vi "offsetZ.vi"(4 "Low Thres":dbl, 6 "Up Thres":dbl, 10 "Current":dbl[][](array[numeric]), 11 "Previous":dbl[][](array[numeric])) -> (2 "OffsetZ":dbl)   [LabVIEW 2011]
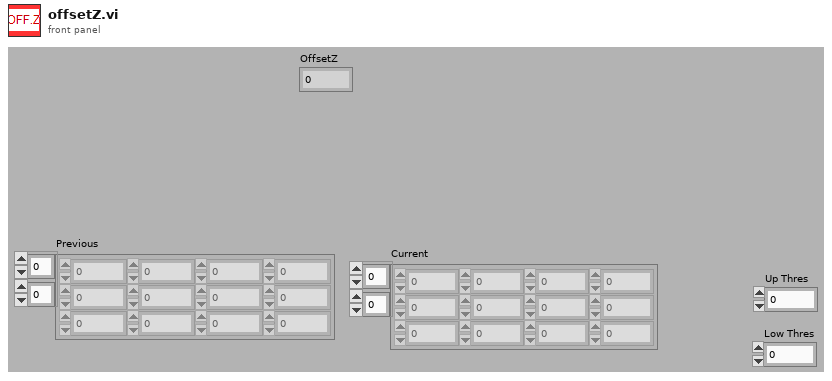
[diagram p1: front panel]
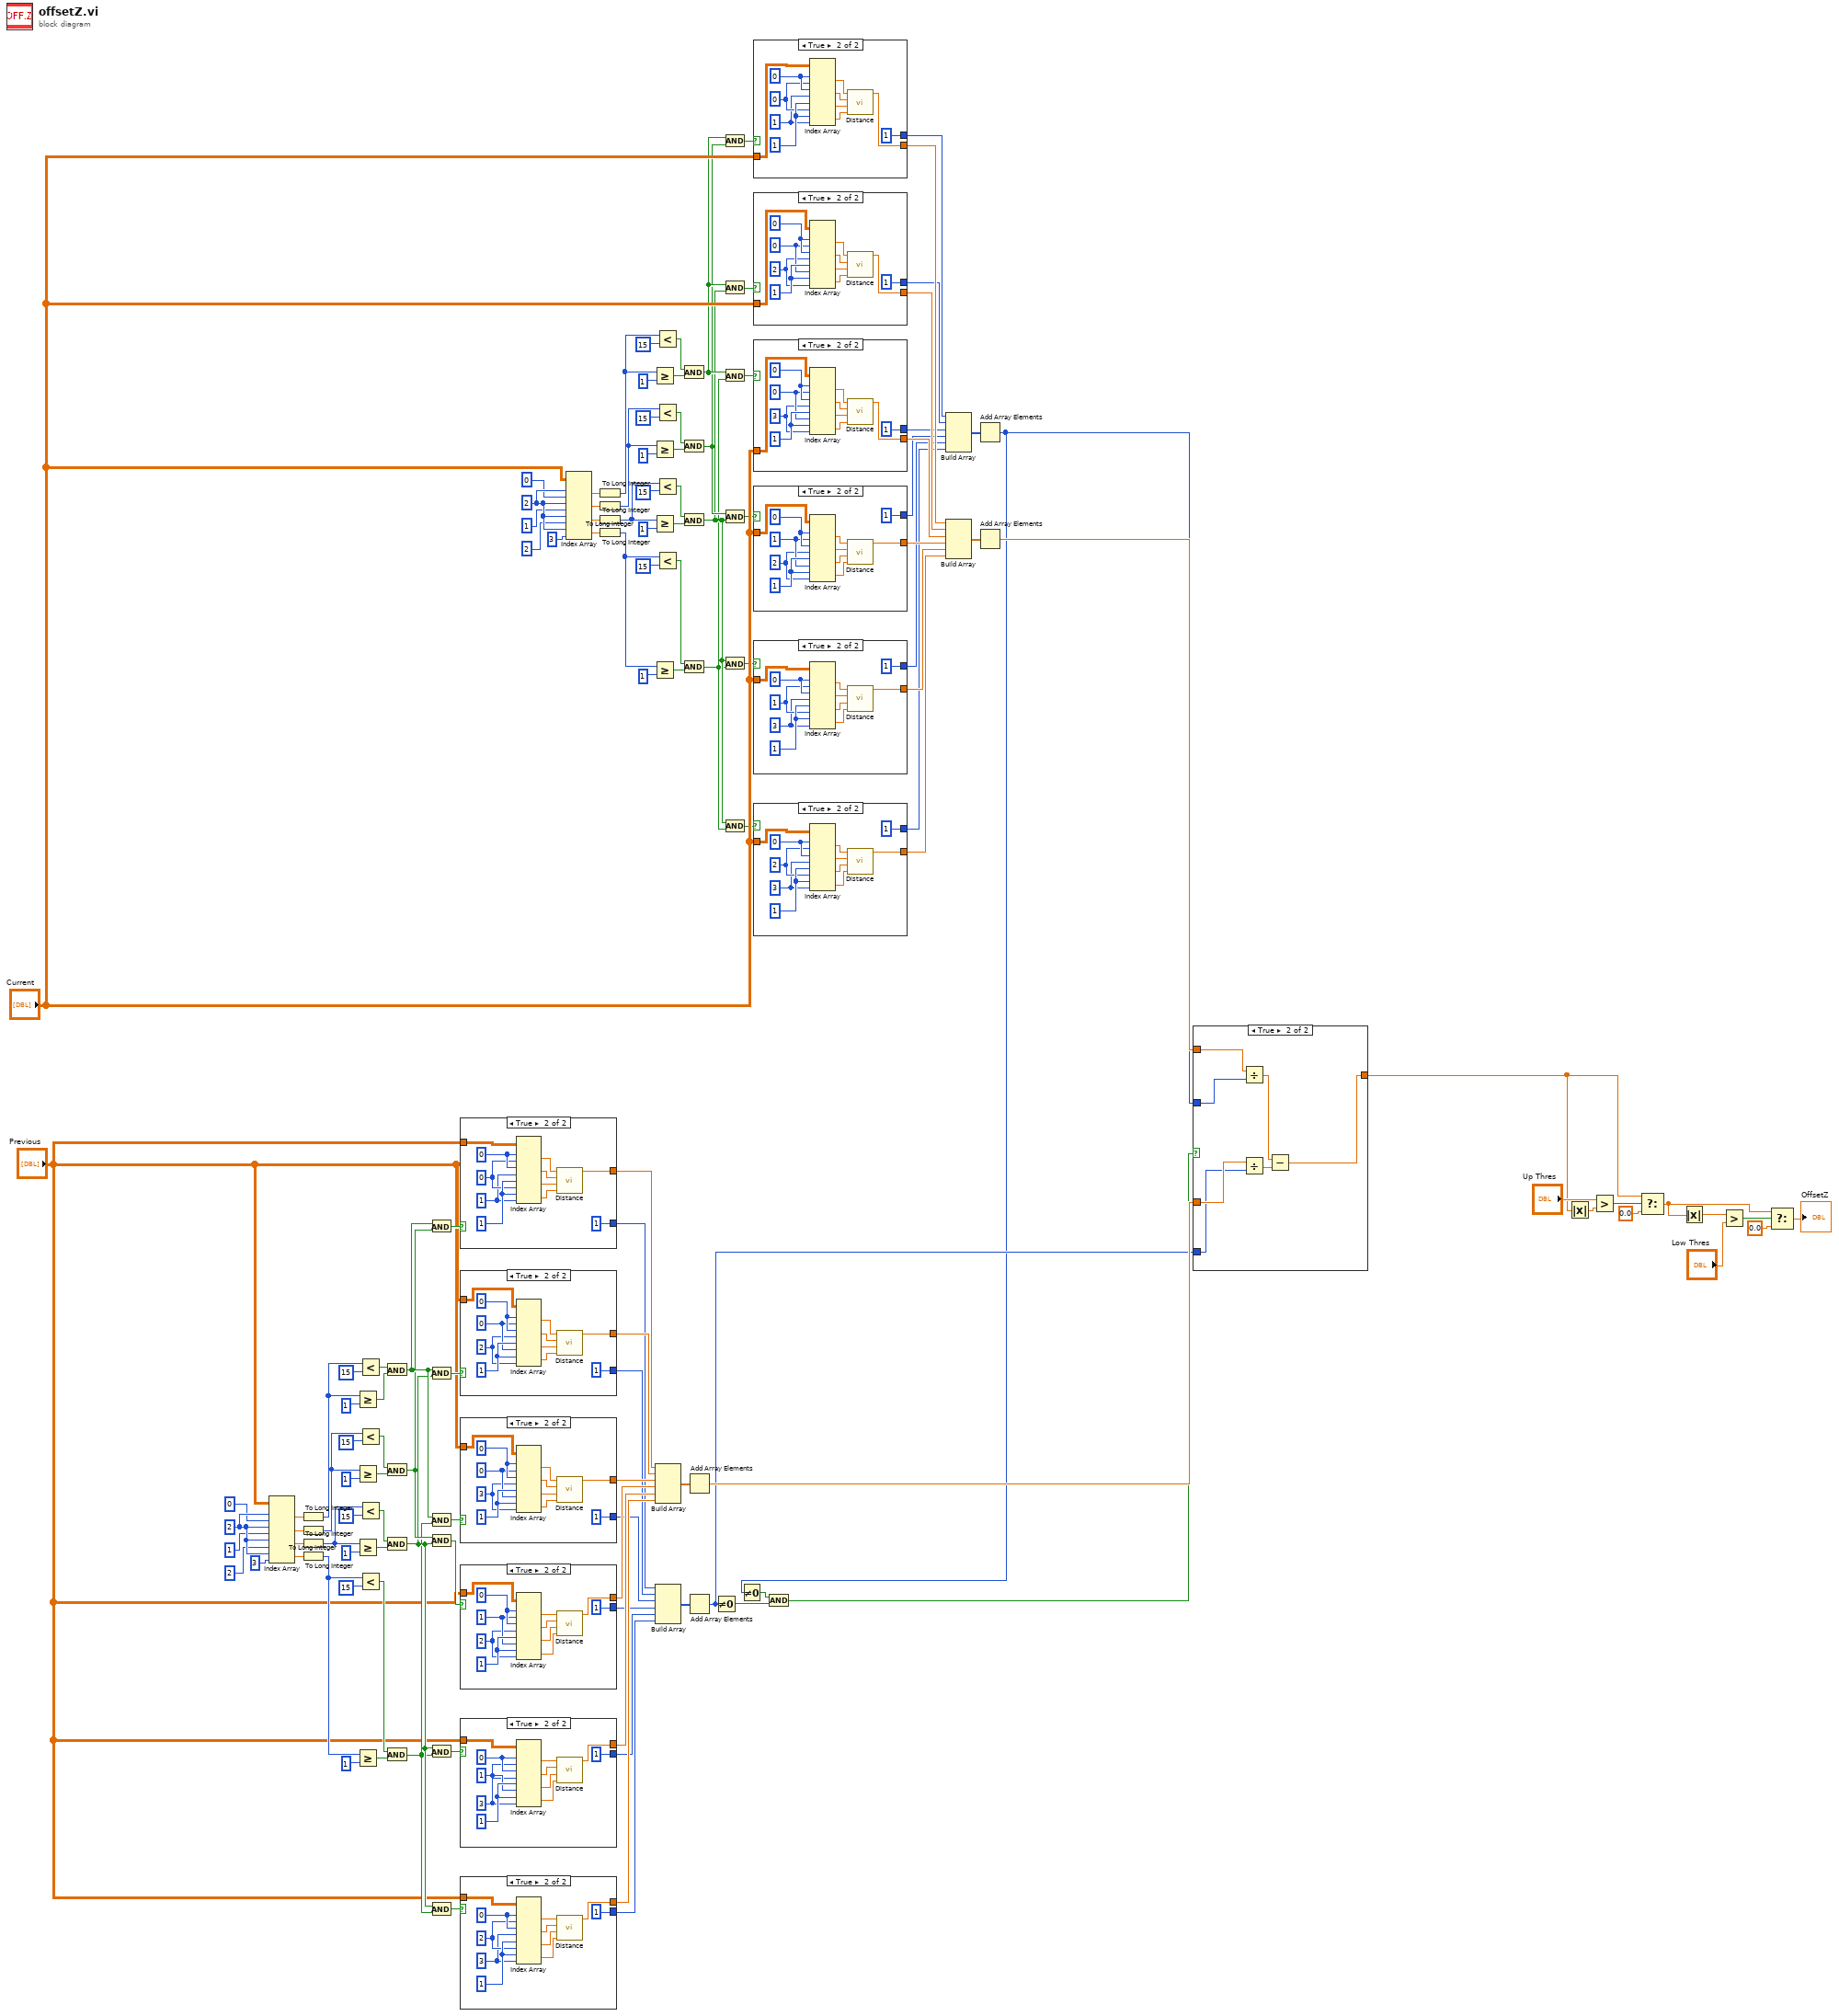
[diagram p0: block diagram]
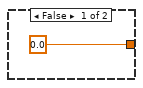
[diagram p2: hidden frame]
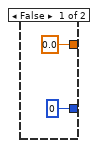
[diagram p3: hidden frame]
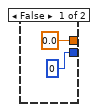
[diagram p4: hidden frame]
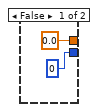
[diagram p5: hidden frame]
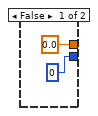
[diagram p6: hidden frame]
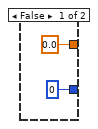
[diagram p7: hidden frame]
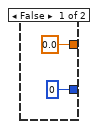
[diagram p8: hidden frame]
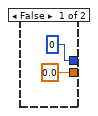
[diagram p9: hidden frame]
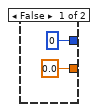
[diagram p10: hidden frame]
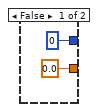
[diagram p11: hidden frame]
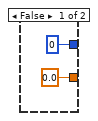
[diagram p12: hidden frame]
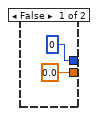
[diagram p13: hidden frame]
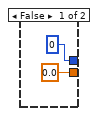
[diagram p14: hidden frame]
diagram:
  w62 = 2 ("index (row)")
  w116 = 2 ("index (row)")
  n1 = Index Array(array="Previous", index (row) #1=w62, index (col) #1=0 ("disabled index (col)"), index (row) #2=w62, index (col) #2=1 ("disabled index (col)"), index (row) #3=w62, index (col) #3=2 ("disabled index (col)"), index (row) #4=w62, index (col) #4=3 ("disabled index (col)")) -> (element #1=w57:dbl, element #2=w56:dbl, element #3=w55:dbl, element #4=w54:dbl)
  n2 = To Long Integer(number=w57) -> (32bit integer=w49:i32)
  n3 = To Long Integer(number=w56) -> (32bit integer=w36:i32)
  n4 = To Long Integer(number=w55) -> (32bit integer=w35:i32)
  n5 = To Long Integer(number=w54) -> (32bit integer=w34:i32)
  n6 = Greater Or Equal?(x=w49, y=1) -> (x >= y?=w50:bool)
  n7 = Greater Or Equal?(x=w36, y=1) -> (x >= y?=w45:bool)
  n8 = Greater Or Equal?(x=w35, y=1) -> (x >= y?=w41:bool)
  n9 = Greater Or Equal?(x=w34, y=1) -> (x >= y?=w37:bool)
  n10 = Less?(x=w49, y=15) -> (x < y?=w51:bool)
  n11 = Less?(x=w36, y=15) -> (x < y?=w46:bool)
  n12 = Less?(x=w35, y=15) -> (x < y?=w42:bool)
  n13 = Less?(x=w34, y=15) -> (x < y?=w38:bool)
  n14 = And(x=w51, y=w50) -> (x .and. y?=w27:bool)
  n15 = And(x=w46, y=w45) -> (x .and. y?=w26:bool)
  n16 = And(x=w42, y=w41) -> (x .and. y?=w25:bool)
  n17 = And(x=w38, y=w37) -> (x .and. y?=w24:bool)
  n18 = And(x=w27, y=w26) -> (x .and. y?=w33:bool)
  n19 = And(x=w27, y=w25) -> (x .and. y?=w32:bool)
  n20 = And(x=w27, y=w24) -> (x .and. y?=w31:bool)
  n21 = And(x=w26, y=w25) -> (x .and. y?=w30:bool)
  n22 = And(x=w25, y=w24) -> (x .and. y?=w29:bool)
  n23 = And(x=w25, y=w24) -> (x .and. y?=w28:bool)
  n24 = case shown="True" w33 {
    tunnel: "Previous" -> [_ w131]
    tunnel: [0.0 ("Dist") w130] -> w23
    tunnel: [0 ("y") 1 ("y")] -> w16
    frame False {
    }
    frame True {
      w132 = 1 ("disabled index (col)")
      w133 = 0 ("disabled index (col)")
      w134 = 1 ("index (row)")
      w135 = 0 ("index (row)")
      n25 = Index Array(array=w131, index (row) #1=w135, index (col) #1=w133, index (row) #2=w135, index (col) #2=w132, index (row) #3=w134, index (col) #3=w133, index (row) #4=w134, index (col) #4=w132) -> (element #1=w139:dbl, element #2=w138:dbl, element #3=w137:dbl, element #4=w136:dbl)
      n26 = call "Distance.vi"("y2"=w136, "y1"=w137, "x2"=w138, "x1"=w139) -> ("Dist"=w130:dbl)  [unwired: 7 in]
    }
  }
  n27 = case shown="True" w32 {
    tunnel: "Previous" -> [_ w144]
    tunnel: [0.0 ("Dist") w143] -> w22
    tunnel: [0 ("y") 1 ("y")] -> w15
    frame False {
    }
    frame True {
      w145 = 2 ("disabled index (col)")
      w146 = 0 ("disabled index (col)")
      w147 = 1 ("index (row)")
      w148 = 0 ("index (row)")
      n28 = Index Array(array=w144, index (row) #1=w148, index (col) #1=w146, index (row) #2=w148, index (col) #2=w145, index (row) #3=w147, index (col) #3=w146, index (row) #4=w147, index (col) #4=w145) -> (element #1=w152:dbl, element #2=w151:dbl, element #3=w150:dbl, element #4=w149:dbl)
      n29 = call "Distance.vi"("y2"=w149, "y1"=w150, "x2"=w151, "x1"=w152) -> ("Dist"=w143:dbl)  [unwired: 7 in]
    }
  }
  n30 = case shown="True" w31 {
    tunnel: "Previous" -> [_ w157]
    tunnel: [0.0 ("Dist") w156] -> w21
    tunnel: [0 ("y") 1 ("y")] -> w14
    frame False {
    }
    frame True {
      w158 = 3 ("disabled index (col)")
      w159 = 0 ("disabled index (col)")
      w160 = 1 ("index (row)")
      w161 = 0 ("index (row)")
      n31 = Index Array(array=w157, index (row) #1=w161, index (col) #1=w159, index (row) #2=w161, index (col) #2=w158, index (row) #3=w160, index (col) #3=w159, index (row) #4=w160, index (col) #4=w158) -> (element #1=w165:dbl, element #2=w164:dbl, element #3=w163:dbl, element #4=w162:dbl)
      n32 = call "Distance.vi"("y2"=w162, "y1"=w163, "x2"=w164, "x1"=w165) -> ("Dist"=w156:dbl)  [unwired: 7 in]
    }
  }
  n33 = case shown="True" w30 {
    tunnel: "Previous" -> [_ w170]
    tunnel: [0.0 ("Dist") w169] -> w20
    tunnel: [0 ("y") 1 ("y")] -> w13
    frame False {
    }
    frame True {
      w171 = 2 ("disabled index (col)")
      w172 = 1 ("disabled index (col)")
      w173 = 1 ("index (row)")
      w174 = 0 ("index (row)")
      n34 = Index Array(array=w170, index (row) #1=w174, index (col) #1=w172, index (row) #2=w174, index (col) #2=w171, index (row) #3=w173, index (col) #3=w172, index (row) #4=w173, index (col) #4=w171) -> (element #1=w178:dbl, element #2=w177:dbl, element #3=w176:dbl, element #4=w175:dbl)
      n35 = call "Distance.vi"("y2"=w175, "y1"=w176, "x2"=w177, "x1"=w178) -> ("Dist"=w169:dbl)  [unwired: 7 in]
    }
  }
  n36 = case shown="True" w29 {
    tunnel: "Previous" -> [_ w183]
    tunnel: [0.0 ("Dist") w182] -> w19
    tunnel: [0 ("y") 1 ("y")] -> w12
    frame False {
    }
    frame True {
      w184 = 3 ("disabled index (col)")
      w185 = 1 ("disabled index (col)")
      w186 = 1 ("index (row)")
      w187 = 0 ("index (row)")
      n37 = Index Array(array=w183, index (row) #1=w187, index (col) #1=w185, index (row) #2=w187, index (col) #2=w184, index (row) #3=w186, index (col) #3=w185, index (row) #4=w186, index (col) #4=w184) -> (element #1=w191:dbl, element #2=w190:dbl, element #3=w189:dbl, element #4=w188:dbl)
      n38 = call "Distance.vi"("y2"=w188, "y1"=w189, "x2"=w190, "x1"=w191) -> ("Dist"=w182:dbl)  [unwired: 7 in]
    }
  }
  n39 = case shown="True" w28 {
    tunnel: "Previous" -> [_ w196]
    tunnel: [0.0 ("Dist") w195] -> w18
    tunnel: [0 ("y") 1 ("y")] -> w11
    frame False {
    }
    frame True {
      w197 = 3 ("disabled index (col)")
      w198 = 2 ("disabled index (col)")
      w199 = 1 ("index (row)")
      w200 = 0 ("index (row)")
      n40 = Index Array(array=w196, index (row) #1=w200, index (col) #1=w198, index (row) #2=w200, index (col) #2=w197, index (row) #3=w199, index (col) #3=w198, index (row) #4=w199, index (col) #4=w197) -> (element #1=w204:dbl, element #2=w203:dbl, element #3=w202:dbl, element #4=w201:dbl)
      n41 = call "Distance.vi"("y2"=w201, "y1"=w202, "x2"=w203, "x1"=w204) -> ("Dist"=w195:dbl)  [unwired: 7 in]
    }
  }
  n42 = Index Array(array="Current", index (row) #1=w116, index (col) #1=0 ("disabled index (col)"), index (row) #2=w116, index (col) #2=1 ("disabled index (col)"), index (row) #3=w116, index (col) #3=2 ("disabled index (col)"), index (row) #4=w116, index (col) #4=3 ("disabled index (col)")) -> (element #1=w111:dbl, element #2=w110:dbl, element #3=w109:dbl, element #4=w108:dbl)
  n43 = To Long Integer(number=w111) -> (32bit integer=w103:i32)
  n44 = To Long Integer(number=w110) -> (32bit integer=w90:i32)
  n45 = To Long Integer(number=w109) -> (32bit integer=w89:i32)
  n46 = To Long Integer(number=w108) -> (32bit integer=w88:i32)
  n47 = Greater Or Equal?(x=w103, y=1) -> (x >= y?=w104:bool)
  n48 = Greater Or Equal?(x=w90, y=1) -> (x >= y?=w99:bool)
  n49 = Greater Or Equal?(x=w89, y=1) -> (x >= y?=w95:bool)
  n50 = Greater Or Equal?(x=w88, y=1) -> (x >= y?=w91:bool)
  n51 = Less?(x=w103, y=15) -> (x < y?=w105:bool)
  n52 = Less?(x=w90, y=15) -> (x < y?=w100:bool)
  n53 = Less?(x=w89, y=15) -> (x < y?=w96:bool)
  n54 = Less?(x=w88, y=15) -> (x < y?=w92:bool)
  n55 = Build Array(w23, w22, w21, w20, w19, w18) -> (w17:dbl[])
  n56 = Build Array(w16, w15, w14, w13, w12, w11) -> (w10:i32[])
  n57 = And(x=w105, y=w104) -> (x .and. y?=w80:bool)
  n58 = And(x=w100, y=w99) -> (x .and. y?=w79:bool)
  n59 = And(x=w96, y=w95) -> (x .and. y?=w78:bool)
  n60 = And(x=w92, y=w91) -> (x .and. y?=w77:bool)
  n61 = Add Array Elements(numeric array=w17) -> (sum=w8:dbl)
  n62 = Add Array Elements(numeric array=w10) -> (sum=w7:i32)
  n63 = Not Equal To 0?(x=w7) -> (x != 0?=w1:bool)
  n64 = And(x=w80, y=w79) -> (x .and. y?=w86:bool)
  n65 = And(x=w80, y=w78) -> (x .and. y?=w85:bool)
  n66 = And(x=w80, y=w77) -> (x .and. y?=w84:bool)
  n67 = And(x=w79, y=w78) -> (x .and. y?=w83:bool)
  n68 = And(x=w78, y=w77) -> (x .and. y?=w82:bool)
  n69 = And(x=w78, y=w77) -> (x .and. y?=w81:bool)
  n70 = case shown="True" w86 {
    tunnel: "Current" -> [_ w209]
    tunnel: [0.0 ("Dist") w208] -> w76
    tunnel: [0 ("y") 1 ("y")] -> w69
    frame False {
    }
    frame True {
      w210 = 1 ("disabled index (col)")
      w211 = 0 ("disabled index (col)")
      w212 = 1 ("index (row)")
      w213 = 0 ("index (row)")
      n71 = Index Array(array=w209, index (row) #1=w213, index (col) #1=w211, index (row) #2=w213, index (col) #2=w210, index (row) #3=w212, index (col) #3=w211, index (row) #4=w212, index (col) #4=w210) -> (element #1=w217:dbl, element #2=w216:dbl, element #3=w215:dbl, element #4=w214:dbl)
      n72 = call "Distance.vi"("y2"=w214, "y1"=w215, "x2"=w216, "x1"=w217) -> ("Dist"=w208:dbl)  [unwired: 7 in]
    }
  }
  n73 = case shown="True" w85 {
    tunnel: "Current" -> [_ w222]
    tunnel: [0.0 ("Dist") w221] -> w75
    tunnel: [0 ("y") 1 ("y")] -> w68
    frame False {
    }
    frame True {
      w223 = 2 ("disabled index (col)")
      w224 = 0 ("disabled index (col)")
      w225 = 1 ("index (row)")
      w226 = 0 ("index (row)")
      n74 = Index Array(array=w222, index (row) #1=w226, index (col) #1=w224, index (row) #2=w226, index (col) #2=w223, index (row) #3=w225, index (col) #3=w224, index (row) #4=w225, index (col) #4=w223) -> (element #1=w230:dbl, element #2=w229:dbl, element #3=w228:dbl, element #4=w227:dbl)
      n75 = call "Distance.vi"("y2"=w227, "y1"=w228, "x2"=w229, "x1"=w230) -> ("Dist"=w221:dbl)  [unwired: 7 in]
    }
  }
  n76 = case shown="True" w84 {
    tunnel: "Current" -> [_ w235]
    tunnel: [0.0 ("Dist") w234] -> w74
    tunnel: [0 ("y") 1 ("y")] -> w67
    frame False {
    }
    frame True {
      w236 = 3 ("disabled index (col)")
      w237 = 0 ("disabled index (col)")
      w238 = 1 ("index (row)")
      w239 = 0 ("index (row)")
      n77 = Index Array(array=w235, index (row) #1=w239, index (col) #1=w237, index (row) #2=w239, index (col) #2=w236, index (row) #3=w238, index (col) #3=w237, index (row) #4=w238, index (col) #4=w236) -> (element #1=w243:dbl, element #2=w242:dbl, element #3=w241:dbl, element #4=w240:dbl)
      n78 = call "Distance.vi"("y2"=w240, "y1"=w241, "x2"=w242, "x1"=w243) -> ("Dist"=w234:dbl)  [unwired: 7 in]
    }
  }
  n79 = case shown="True" w83 {
    tunnel: "Current" -> [_ w248]
    tunnel: [0.0 ("Dist") w247] -> w73
    tunnel: [0 ("y") 1 ("y")] -> w66
    frame False {
    }
    frame True {
      w249 = 2 ("disabled index (col)")
      w250 = 1 ("disabled index (col)")
      w251 = 1 ("index (row)")
      w252 = 0 ("index (row)")
      n80 = Index Array(array=w248, index (row) #1=w252, index (col) #1=w250, index (row) #2=w252, index (col) #2=w249, index (row) #3=w251, index (col) #3=w250, index (row) #4=w251, index (col) #4=w249) -> (element #1=w256:dbl, element #2=w255:dbl, element #3=w254:dbl, element #4=w253:dbl)
      n81 = call "Distance.vi"("y2"=w253, "y1"=w254, "x2"=w255, "x1"=w256) -> ("Dist"=w247:dbl)  [unwired: 7 in]
    }
  }
  n82 = case shown="True" w82 {
    tunnel: "Current" -> [_ w261]
    tunnel: [0.0 ("Dist") w260] -> w72
    tunnel: [0 ("y") 1 ("y")] -> w65
    frame False {
    }
    frame True {
      w262 = 3 ("disabled index (col)")
      w263 = 1 ("disabled index (col)")
      w264 = 1 ("index (row)")
      w265 = 0 ("index (row)")
      n83 = Index Array(array=w261, index (row) #1=w265, index (col) #1=w263, index (row) #2=w265, index (col) #2=w262, index (row) #3=w264, index (col) #3=w263, index (row) #4=w264, index (col) #4=w262) -> (element #1=w269:dbl, element #2=w268:dbl, element #3=w267:dbl, element #4=w266:dbl)
      n84 = call "Distance.vi"("y2"=w266, "y1"=w267, "x2"=w268, "x1"=w269) -> ("Dist"=w260:dbl)  [unwired: 7 in]
    }
  }
  n85 = case shown="True" w81 {
    tunnel: "Current" -> [_ w274]
    tunnel: [0.0 ("Dist") w273] -> w71
    tunnel: [0 ("y") 1 ("y")] -> w64
    frame False {
    }
    frame True {
      w275 = 3 ("disabled index (col)")
      w276 = 2 ("disabled index (col)")
      w277 = 1 ("index (row)")
      w278 = 0 ("index (row)")
      n86 = Index Array(array=w274, index (row) #1=w278, index (col) #1=w276, index (row) #2=w278, index (col) #2=w275, index (row) #3=w277, index (col) #3=w276, index (row) #4=w277, index (col) #4=w275) -> (element #1=w282:dbl, element #2=w281:dbl, element #3=w280:dbl, element #4=w279:dbl)
      n87 = call "Distance.vi"("y2"=w279, "y1"=w280, "x2"=w281, "x1"=w282) -> ("Dist"=w273:dbl)  [unwired: 7 in]
    }
  }
  n88 = Build Array(w69, w68, w67, w66, w65, w64) -> (w63:i32[])
  n89 = Build Array(w76, w75, w74, w73, w72, w71) -> (w70:dbl[])
  n90 = Add Array Elements(numeric array=w63) -> (sum=w5:i32)
  n91 = Not Equal To 0?(x=w5) -> (x != 0?=w2:bool)
  n92 = And(x=w2, y=w1) -> (x .and. y?=w3:bool)
  n93 = Add Array Elements(numeric array=w70) -> (sum=w6:dbl)
  n94 = case shown="True" w3 {
    tunnel: w5 -> [_ w290]
    tunnel: w6 -> [_ w289]
    tunnel: [0.0 w284] -> w4
    tunnel: w8 -> [_ w288]
    tunnel: w7 -> [_ w287]
    frame False {
    }
    frame True {
      n95 = Divide(x=w289, y=w290) -> (x/y=w285:dbl)
      n96 = Divide(x=w288, y=w287) -> (x/y=w286:dbl)
      n97 = Subtract(x=w285, y=w286) -> (x-y=w284:dbl)
    }
  }
  n98 = Absolute Value(x=w4) -> (abs(x)=w125:dbl)
  n99 = Greater?(x="Up Thres", y=w125) -> (0:w126:bool)
  n100 = Select(t=w4, s=w126, f=0.0) -> (s? t:f=w120:dbl)
  n101 = Absolute Value(x=w120) -> (abs(x)=w119:dbl)
  n102 = Greater?(x=w119, y="Low Thres") -> (0:w122:bool)
  n103 = Select(t=w120, s=w122, f=0.0) -> (s? t:f=→"OffsetZ":dbl)
